vi "LJ_Handles_Global.vi"() -> ()   [LabVIEW 2016]
panel:
  in  "LJ Handles":i32[](array[numeric])
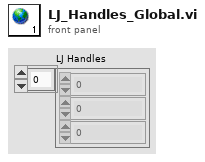
[diagram p1: front panel]
diagram:
